vi "test udp r-2.vi"() -> ()   [LabVIEW 2019]
panel:
  out "웨이브폼 그래프":u8[][](graph)
  out "포트":u16
  in  "Stop":bool
  out "데이터 출력":string
  out "숫자형":i32=151
  out "주소":u32
  in  "대기 시간 (ms)":u32=50
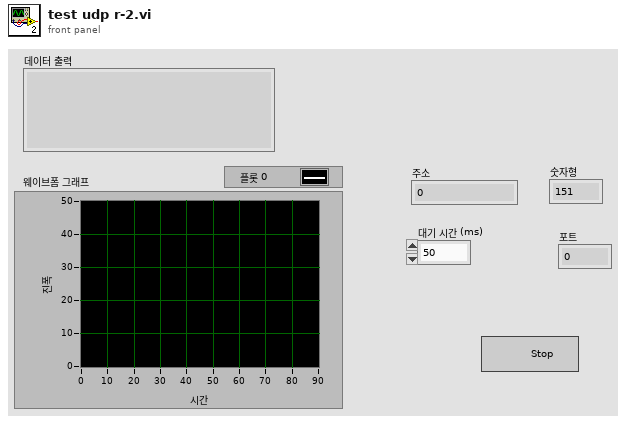
[diagram p1: front panel]
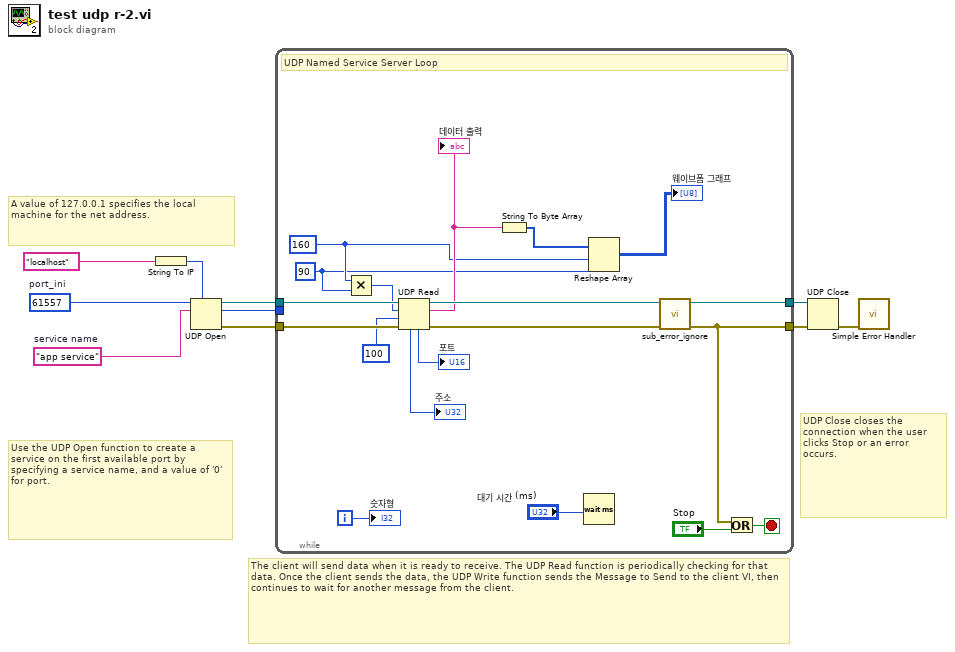
[diagram p0: block diagram]
diagram:
  w1 = u16 61557  # port_ini
  w10 = "app service"  # service name
  # "UDP Close closes the connection when the user clicks Stop or an error occurs."
  # "A value of 127.0.0.1 specifies the local machine for the net address."
  # "The client will send data when it is ready to receive. The UDP Read function is periodically checking for that data. Once the client sends the data, the UDP Write function sends the Message to Send to the client VI, then continues to wait for another message from the client."
  # "Use the UDP Open function to create a service on the first available port by specifying a service name, and a value of '0' for port."
  n1 = String To IP(1:"localhost") -> (0:w5:u32)
  n2 = UDP Open(7:w5, 10:w10, 11:w1) -> (port=w9:refnum<k16>, 0:w8:errorcluster, 2:w3:u16)  [unwired: 2 in]
  n3 = while {
    tunnel: [w18] -> w6
    tunnel: w9 -> [w28]
    tunnel: w8 -> [w27]
    tunnel: [w20] -> w7
    tunnel: w3 -> [_]
    i -> [w22]
    stop <- w26 stop-if-true
    w11 = 90 ("차원 크기")
    w12 = 160 ("차원 크기")
    # "UDP Named Service Server Loop"
    n4 = Multiply(x=w12, y=w11) -> (x*y=w13:i32)
    n5 = UDP Read(connection ID=w28, max size (548)=w13, timeout ms (25000)=100, 8:w27) -> (data out=w16:string, error out=w19:errorcluster, 3:w20:refnum<k16>, 4:→"포트":u16, 6:→"주소":u32)
    "데이터 출력" <- w16
    n6 = String To Byte Array(string=w16) -> (unsigned byte array=w15:u8[])
    n7 = Wait (ms)(milliseconds to wait="대기 시간 (ms)") -> ()  [unwired: 1 out]
    n8 = Reshape Array(w15, w12, w11) -> (→"웨이브폼 그래프":u8[][])
    n9 = call "sub_error_ignore.vi"("error in"=w19) -> ("error out"=w18:errorcluster)  [unwired: 10 in]
    n10 = Or(x=w18, y="Stop") -> (x .or. y?=w26:bool)
    "숫자형" <- w22
  }
  n11 = UDP Close(connection ID=w7, 8:w6) -> (error out=w2:errorcluster)  [unwired: 1 out]
  n12 = call <vilib>:"Simple Error Handler.vi"("error in (no error)"=w2) -> ()  [unwired: 4 in, 5 out]
